vi "Robot_s Second Move.vi"(0 "VISA Refnum in":refnum<visa-resource-name>="COM6", 5 "Index from First Move":u8, 9 "In Play Array":i32[](array[numeric])=[1, 1, 1, 1, 1, 1, 1, 1, 1, 1, 1, 1, 1, 1, 1, 1, 1, 1], 11 "Current Image Array":i32[](array[numeric])=[1, 1, 1, 1, 1, 1, 1, 1, 1, 1, 1, 1, 1, 1, 1, 1, 1, 1]) -> (4 "VISA Refnum out":refnum<visa-resource-name>, 6 "Output Image Array":i32[](array[numeric]), 8 "error out":errorcluster, 10 "Image Value from Second Turn":i32, 15 "Index From Second Move":i32)   [LabVIEW 2018]
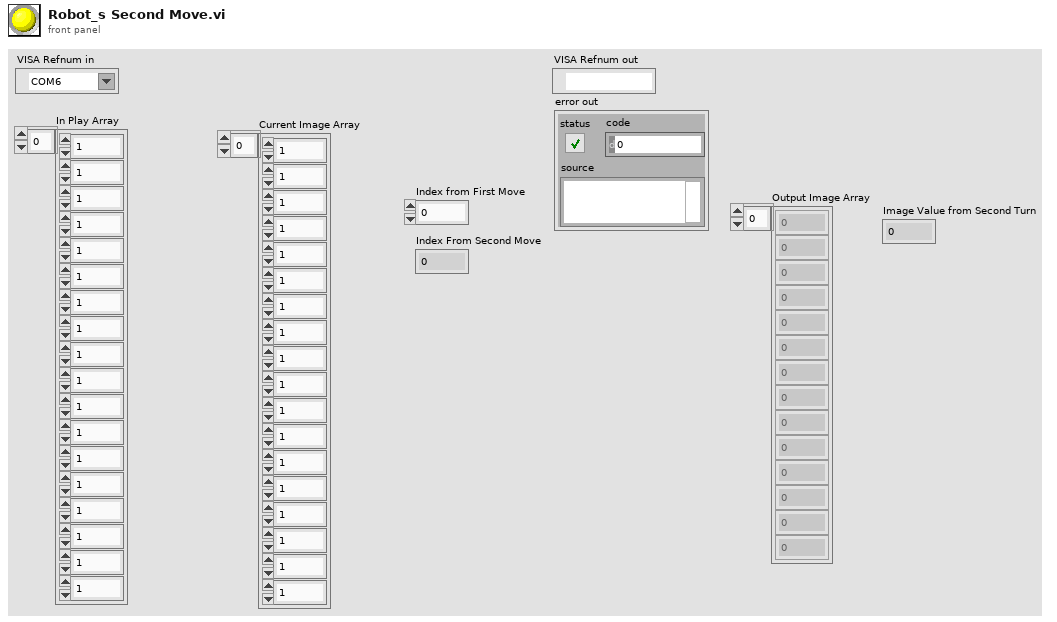
[diagram p1: front panel]
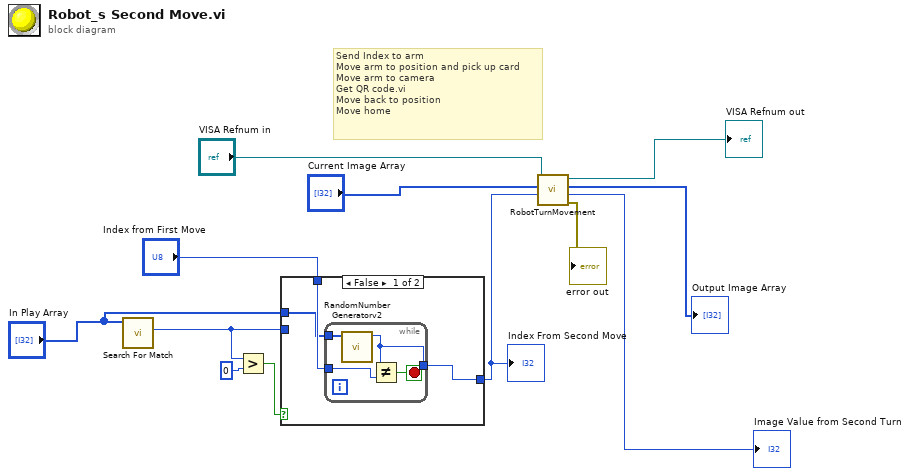
[diagram p0: block diagram]
diagram:
  # "Send Index to arm\nMove arm to position and pick up card\nMove arm to camera\nGet QR code.vi\nMove back to position\nMove home"
  n1 = call "Search For Match.vi"("Array"="In Play Array") -> ("Index 2"=w9:i32)  [unwired: 9 in, 1 out]
  n2 = Greater?(x=w9, y=0) -> (0:w10:bool)
  n3 = case shown="False" w10 {
    tunnel: [w15 w20] -> w6
    tunnel: w9 -> [_ w20]
    tunnel: "Index from First Move" -> [w14 _]
    tunnel: "In Play Array" -> [w13 _]
    frame False {
      n4 = while {
        tunnel: [w18] -> w15
        tunnel: w14 -> [w17]
        tunnel: w13 -> [w16]
        stop <- w19 stop-if-true
        n5 = call "RandomNumberGeneratorv2.vi"("In Play Array"=w16) -> ("Index"=w18:u8)  [unwired: 10 in]
        n6 = Not Equal?(x=w18, y=w17) -> (x != y?=w19:bool)
      }
    }
    frame True {
    }
  }
  "Index From Second Move" <- w6
  n7 = call "RobotTurnMovement.vi"("index"=w6, "Current Image Array"="Current Image Array", "VISA Refnum in"="VISA Refnum in") -> ("error out"=→"error out":errorcluster, "Image Value"=→"Image Value from Second Turn":i32, "Output Array"=→"Output Image Array":i32[], "VISA Refnum out"=→"VISA Refnum out":refnum<visa-resource-name>)  [unwired: 5 in]
